vi "RSZVB Acquire Source Power Calibration.vi"(7 "Port Number (1)":i32=1, 8 "error in (no error)":errorcluster {"code" format="%.0x"}, 9 "Source (0: Port)":i32(ring) items=["Port", "Generator", "Converter"], 10 "Channel (1)":i32=1, 11 "VISA session":refnum<visa-resource-name>) -> (0 "error out":errorcluster {"code" format="%.0x"}, 3 "dup VISA session":refnum<visa-resource-name>)   [LabVIEW 2011]
doc: "This VI selects the source for the source power calibration, starts and applies the source power calibration.\n\nNote(s):\n\n(1) The VI cannot be used unless a power meter is connected via GPIB bus, USB or LAN interface and configured in the System - System Config - Configure External Power Meter\n\n(2) For some measurements the default set timeout can be insufficient. To set higher timeout use VI RSZVB Set Time Out.vi.\n\nRemote-control command(s):\nSOURce<Ch>:POWer<Pt>:CORRection[:ACQuire] PORT | GENerator | CONVerter,<port_number>"
uses:
  _utility/RSZVB Global Data.vi
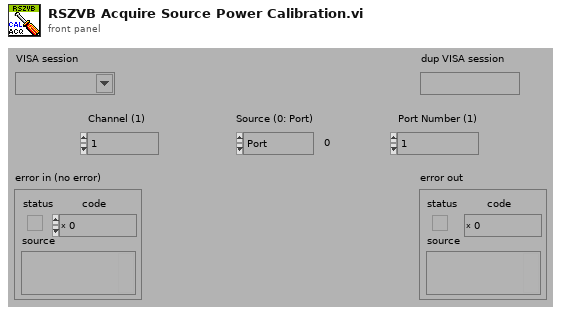
[diagram p1: front panel]
types:
  T1 = cluster{"Error Checking (T: On)":bool, "Installed Options":string[], "Data Valid?":bool, "Ports":i32, "Model":string[], "Option Checking (T: On)":bool}[]
  T2 = cluster{"Error Checking (T: On)":bool, "Installed Options":string[], "Data Valid?":bool, "Ports":i32, "Model":string[], "Option Checking (T: On)":bool}
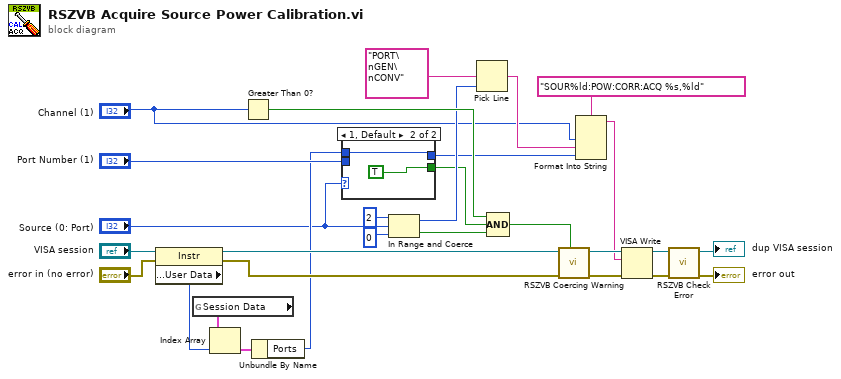
[diagram p0: block diagram]
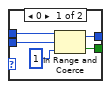
[diagram p2: hidden frame]
diagram:
  n1 = property class="Instr"(reference="VISA session", error in="error in (no error)") -> (reference out=w12:refnum<visa-resource-name>, error out=w13:errorcluster, "General Settings:User Data"=w14:u32)
  n2 = global read "RSZVB Global Data.vi" "Session Data"() -> (w15:T1)
  n3 = Index Array(array=w15, index=w14) -> (element=w16:T2)
  n4 = Greater Than 0?(x="Channel (1)") -> (x > 0?=w24:bool)
  n5 = Unbundle By Name(w16) -> ("Ports"=w7:i32)
  n6 = case shown="1, Default" "Source (0: Port)" {
    tunnel: [w30 w35] -> w9
    tunnel: "Port Number (1)" -> [w33 _]
    tunnel: w7 -> [w32 w35]
    tunnel: [w31 TRUE] -> w6
    frame 0 {
      n7 = In Range and Coerce(upper limit=w32, x=w33, lower limit=1) -> (coerced(x)=w30:i32, In Range?=w31:bool)
    }
    frame 1, Default {
    }
  }
  n8 = In Range and Coerce(upper limit=2, x="Source (0: Port)", lower limit=0) -> (coerced(x)=w19:i32, In Range?=w17:bool)
  n9 = Pick Line(multi-line string="PORT\nGEN\nCONV", line index=w19) -> (output string=w3:string)  [unwired: 1 in]
  n10 = Compound Arithmetic op=AND(w24, w6, w17) -> (w23:bool)
  n11 = call "RSZVB Coercing Warning.vi"("In Range?"=w23, "error in (no error)"=w13, "VISA session"=w12) -> ("error out"=w5:errorcluster, "dup VISA session"=w27:refnum<visa-resource-name>)  [unwired: 7 in]
  n12 = Format Into String(format string="SOUR%ld:POW:CORR:ACQ %s,%ld", "Channel (1)", w3, w9) -> (resulting string=w22:string)  [unwired: 2 in, 1 out]
  n13 = VISA Write(VISA resource name=w27, write buffer=w22, error in (no error)=w5) -> (VISA resource name out=w25:refnum<visa-resource-name>, error out=w26:errorcluster)  [unwired: 1 out]
  n14 = call "RSZVB Check Error.vi"("error in (no error)"=w26, "VISA session"=w25) -> ("error out"=→"error out":errorcluster, "dup VISA session"=→"dup VISA session":refnum<visa-resource-name>)  [unwired: 8 in]
